vi "TestStimTiming.vi"() -> ()   [LabVIEW 2017]
uses:
  <vilib>/Platform/TimedLoop/XDataNode/timing_clust.ctl
  <vilib>/Platform/TimedLoop/XDataNode/nitl_modes.ctl
  <vilib>/Platform/TimedLoop/XDataNode/wakeup.ctl
  <vilib>/DAQmx/write.llb/DAQmx Write (Digital Bool 1Line 1Point).vi
  <vilib>/Platform/TimedLoop/scheduler/LVUserAPI/_suppVIs/Create_1kHz_TSource.vi
  <vilib>/DAQmx/create/timing.llb/DAQmx Create Timing Source (Digital Edge using Counter).vi
  <vilib>/DAQmx/miscellaneous.llb/DAQmx Fill In Error Info.vi
  <vilib>/platform/TimedLoop/XDataNode/XDataNode.xnode
  <vilib>/Platform/TimedLoop/XDataNode/XDNodeRunTimeDep.lvlib
panel:
  in  "Use sample clock\nfrom OEP board":bool
  out "error out":errorcluster
  in  "Stop Button":bool
  in  "Period (ms)":i64=200
  in  "DO Physical channel":tag="pciDAQ/port0/line7"
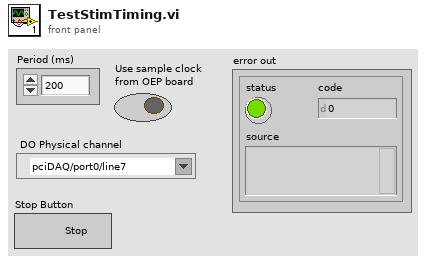
[diagram p1: front panel]
types:
  T1 = typedef "XDNodeRunTimeDep.lvlib/timing_clust.ctl" = cluster{"Expected End [f-1]":u64, "Actual End [f-1]":u64, "Finished Late? [f-1]":bool, "Expected End [i-1]":u64, "Actual End [i-1]":u64, "Finished Late? [i-1]":bool, "Expected Start [i]":u64, "Actual Start [i]":u64, "Expected Start [f]":u64, "Actual Start [f]":u64, "Source Name":string, "Structure Name":string, "Period":i64, "Deadline":i64, "Offset":i64, "Start":i64, "Priority":i32, "Timeout":i32, "Mode":T2, "Wakeup Reason":T3, "Error":errorcluster, "Source Type":string, "Secondary Source Type":string, "Global End Time":u64, "Global Start Time":u64, "Frame Duration":u64, "Iteration Duration":u64, "Assigned CPU":i32, "I/O Scan Engine Mode":u32}
  T2 = typedef "XDNodeRunTimeDep.lvlib/nitl_modes.ctl" = enum32{"No Change", "Process missed periods, maintain original phase", "Discard missed periods, maintain original phase", "Process missed periods, ignore original phase", "Discard missed periods, ignore original phase"}
  T3 = typedef "XDNodeRunTimeDep.lvlib/wakeup.ctl" = enum32{"Normal", "Aborted", "Asynchronous wakeup", "Timing source error", "Timed loop error", "Timeout"}
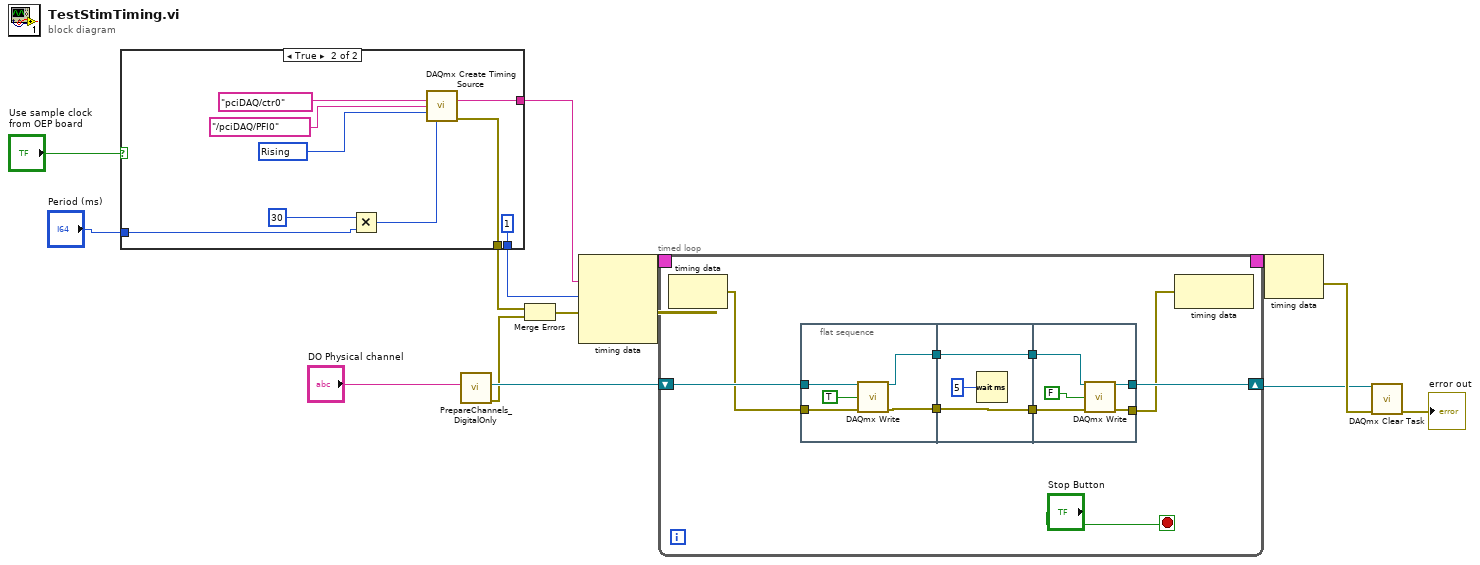
[diagram p0: block diagram]
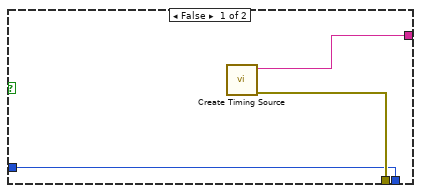
[diagram p2: hidden frame]
diagram:
  n1 = case shown="True" "Use sample clock\nfrom OEP board" {
    tunnel: [w16 w26] -> w5
    tunnel: [w17 w22] -> w4
    tunnel: [w15 i64 1] -> w2
    tunnel: "Period (ms)" -> [w15 w20]
    frame False {
      n2 = call-poly <vilib>:"Create Timing Source.vi"() -> ("error out"=w17:errorcluster, "name (out)"=w16:string)  [unwired: 10 in]
    }
    frame True {
      w24 = 10280 items=["Rising"=10280, "Falling"=10171] ("edge")
      n3 = Multiply(x=i64 30, y=w20) -> (x*y=w18:i64)
      n4 = call-poly <vilib>:"DAQmx Create Timing Source.vi"("counter"=tag "pciDAQ/ctr0", "source"=tag "/pciDAQ/PFI0" ("OEP sample clock in"), "edge"=w24, "edge count"=w18) -> ("timing source out"=w26:string, "error out"=w22:errorcluster)  [unwired: 10 in]
    }
  }
  n5 = call "PrepareChannels_DigitalOnly.vi"("DO Physical channels"="DO Physical channel") -> ("DO task out"=w12:refnum<k21>, "DO error out"=w9:errorcluster)  [unwired: 8 in]
  n6 = Merge Errors(w4, w9) -> (w10:errorcluster)
  n7 = node-c288(w5, w2, w10) -> (w14:T1)  [unwired: 1 in]
  n8 = timed-loop {
    timing: w14 -> [_]
    timing-out: [_] -> w13
    shift-right: [w29] -> w7
    shift-left: w12 -> [w30]
    stop <- "Stop Button" stop-if-true
    n9 = node-c288() -> (w27:errorcluster)  [unwired: 1 in]
    n10 = flat-sequence {
      tunnel: [w40] -> w34
      tunnel: [w38] -> w33
      tunnel: w30 -> [w37]
      tunnel: w27 -> [w36]
      tunnel: [w43] -> w32
      tunnel: w34 -> [w43]
      tunnel: [w41] -> w31
      tunnel: w33 -> [w41]
      tunnel: w32 -> [w48]
      tunnel: [w47] -> w28
      tunnel: w31 -> [w45]
      tunnel: [w44] -> w29
      frame #0 {
        n11 = call-poly <vilib>:"DAQmx Write.vi"("task/channels in"=w37, "data"=TRUE, "error in"=w36) -> ("task out"=w38:refnum<k21>, "error out"=w40:errorcluster)  [unwired: 10 in, 1 out]
      }
      frame #1 {
        n12 = Wait (ms)(milliseconds to wait=u32 5) -> ()  [unwired: 1 out]
      }
      frame #2 {
        n13 = call-poly <vilib>:"DAQmx Write.vi"("task/channels in"=w45, "data"=FALSE, "error in"=w48) -> ("task out"=w44:refnum<k21>, "error out"=w47:errorcluster)  [unwired: 10 in, 1 out]
      }
    }
    n14 = node-c288(w28) -> ()  [unwired: 1 out]
  }
  n15 = node-c288(w13) -> (w8:errorcluster)
  n16 = call <vilib>:"DAQmx Clear Task.vi"("task in"=w7, "error in"=w8) -> ("error out"=→"error out":errorcluster)  [unwired: 13 in]
